vi "FPS control.vi"(3 "error in (no error)":errorcluster) -> (0 "error out":errorcluster, 2 "FPS out":u32)   [LabVIEW 2012]
panel:
  in  "OK Button":bool
  in  "FPS in":u32
  # "Введите частоту кадров (FPS)\n анализируемого видео"
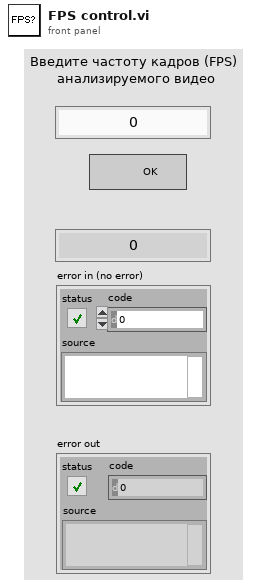
[diagram p1: front panel]
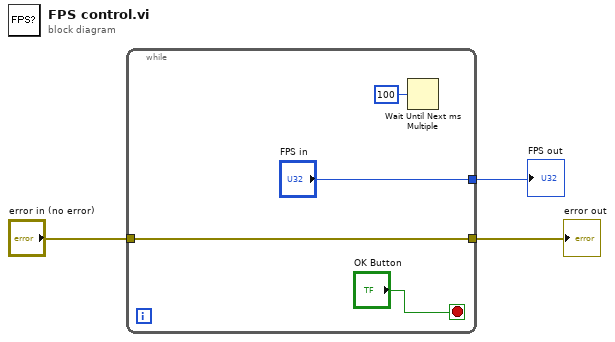
[diagram p0: block diagram]
diagram:
  n1 = while {
    tunnel: ["FPS in"] -> w3
    tunnel: [w4] -> w2
    tunnel: "error in (no error)" -> [w4]
    stop <- "OK Button" stop-if-true
    n2 = Wait Until Next ms Multiple(millisecond multiple=u32 100) -> ()  [unwired: 1 out]
  }
  "FPS out" <- w3
  "error out" <- w2
